vi "Match_fids_by_name.vi"(0 "CurrentSessionDataSet":T1[](array[typedef]), 1 "ReferenceSessionDataSet":T1[](array[typedef])) -> (2 "ReferenceMatch":i32[](array[numeric]), 3 "NumberOfNameMatch":i32, 4 "AtLeast3":bool, 5 "CurrentMatch":i32[](array[numeric]))   [LabVIEW 2011]
doc: "Match fiducials between the reference and current session by name. Determine if there are a minimum of three matching fiducials to calculate the transformation."
uses:
  cm2nm_coordinate_information_v2.ctl
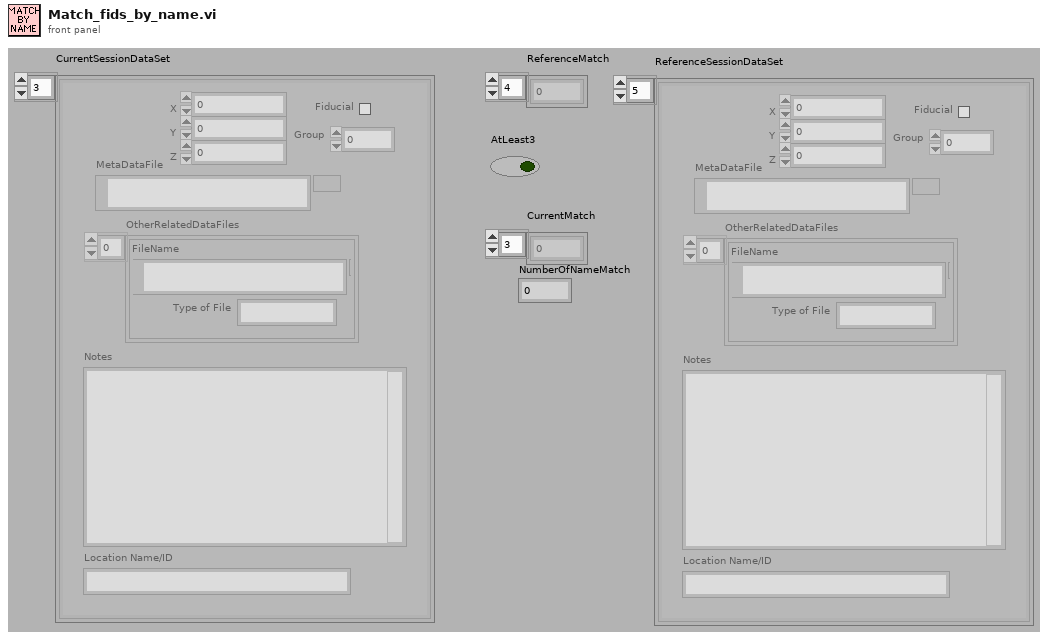
[diagram p1: front panel]
types:
  T1 = typedef "cm2nm_coordinate_information_v2.ctl" = cluster{"MetaDataFile":path, "X":dbl, "Y":dbl, "Z":dbl, "Group":i32, "Rotation":dbl[unit], "Fiducial":bool, "Magnification":dbl, "Working_Distance":dbl, "Notes":string, "Location Name/ID":string, "OtherRelatedDataFiles":cluster{"Type of File":string, "FileName":path}[], "Available":bool}
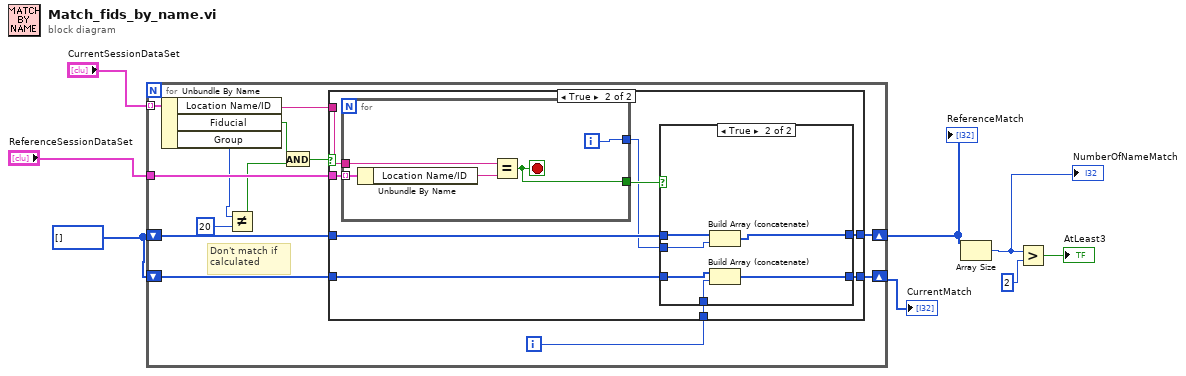
[diagram p0: block diagram]
diagram:
  w3 = i32[] []
  n1 = for {
    tunnel: "CurrentSessionDataSet" -> [w20] mode=indexing
    tunnel: "ReferenceSessionDataSet" -> [w21]
    shift-right: [w17] -> w5
    shift-left: w3 -> [w18]
    shift-right: [w15] -> w4
    shift-left: w3 -> [w16]
    i -> [w14]
    # "Don't match if \ncalculated"
    n2 = Unbundle By Name(w20) -> ("Location Name/ID"=w19:string, "Fiducial"=w10:bool, "Group"=w13:i32)
    n3 = Not Equal?(x=w13, y=20) -> (x != y?=w11:bool)
    n4 = And(x=w10, y=w11) -> (x .and. y?=w9:bool)
    n5 = case shown="True" w9 {
      tunnel: w21 -> [_ w32]
      tunnel: w19 -> [_ w31]
      tunnel: w18 -> [w23 w29]
      tunnel: [w23 w28] -> w17
      tunnel: w16 -> [w22 w27]
      tunnel: [w22 w26] -> w15
      tunnel: w14 -> [_ w25]
      frame False {
      }
      frame True {
        n6 = for {
          tunnel: w32 -> [w45] mode=indexing
          tunnel: w31 -> [w43]
          tunnel: [w42] -> w24
          tunnel: [w41] -> w30
          i -> [w42]
          stop <- w41 stop-if-true
          n7 = Unbundle By Name(w45) -> ("Location Name/ID"=w44:string)
          n8 = Equal?(x=w43, y=w44) -> (x = y?=w41:bool)
        }
        n9 = case shown="True" w30 {
          tunnel: w29 -> [w34 w38]
          tunnel: [w34 w39] -> w28
          tunnel: w27 -> [w33 w37]
          tunnel: [w33 w40] -> w26
          tunnel: w25 -> [_ w36]
          tunnel: w24 -> [_ w35]
          frame False {
          }
          frame True {
            n10 = Build Array (concatenate)(w38, w35) -> (w39:i32[])
            n11 = Build Array (concatenate)(w37, w36) -> (w40:i32[])
          }
        }
      }
    }
  }
  "ReferenceMatch" <- w5
  "CurrentMatch" <- w4
  n12 = Array Size(array=w5) -> (size(s)=w6:i32)
  "NumberOfNameMatch" <- w6
  n13 = Greater?(x=w6, y=2) -> (0:→"AtLeast3":bool)
